vi "执行结果反馈与日志存储.vi"(9 "日志信息":string, 10 "error out":T1, 11 "设备":string) -> ()   [LabVIEW 2016]
panel:
  out "执行结果定义":u16(ring) items=["执行成功"=1, "执行失败，但不知道原因"=2, "命令请求条件错误"=3, "通讯超时"=4, "系统繁忙不能执行"=5, "系统故障"=6, "没有数据"=100]
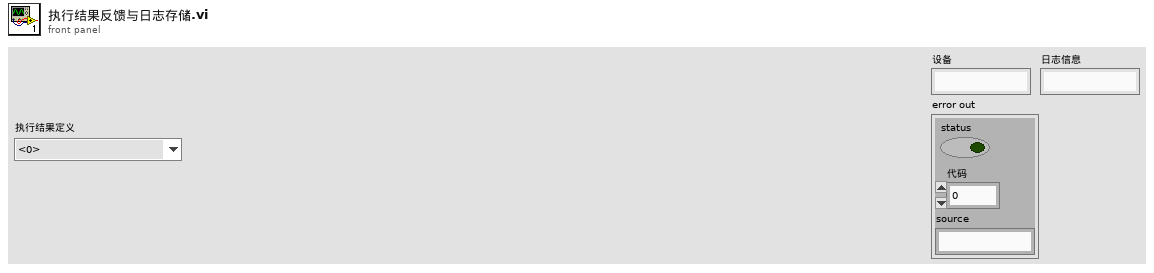
[diagram p1: front panel]
types:
  T1 = cluster{"status":bool, "代码":u16, "source":string}
  T2 = cluster{"时间标识":timestamp, "设备":string, "日志信息":string, "流程参数":string}
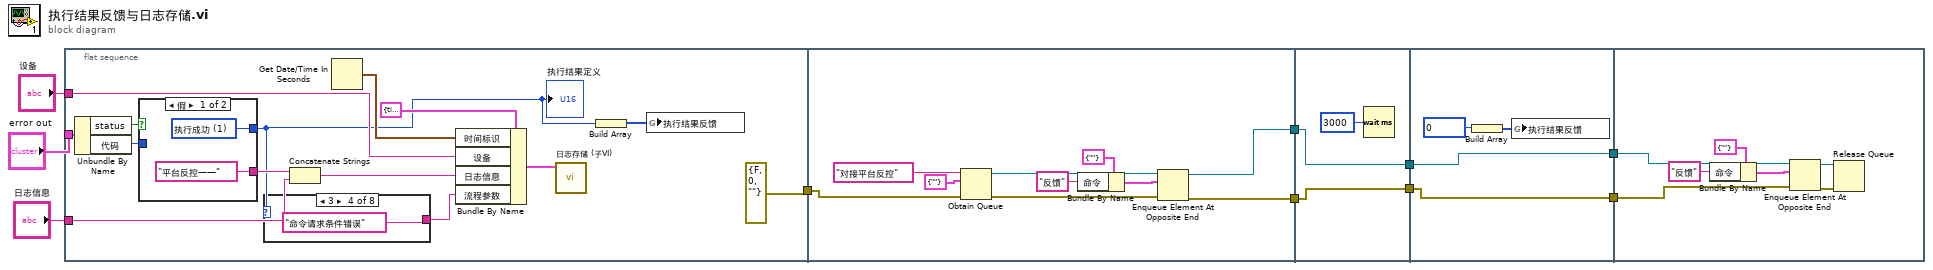
[diagram p0: block diagram]
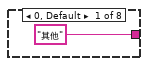
[diagram p2: hidden frame]
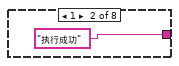
[diagram p3: hidden frame]
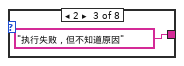
[diagram p4: hidden frame]
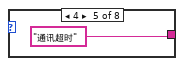
[diagram p5: hidden frame]
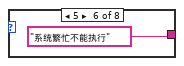
[diagram p6: hidden frame]
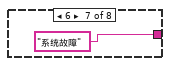
[diagram p7: hidden frame]
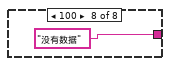
[diagram p8: hidden frame]
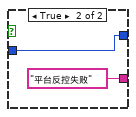
[diagram p9: hidden frame]
diagram:
  n1 = flat-sequence {
    tunnel: "日志信息" -> [w17]
    tunnel: "error out" -> [w16]
    tunnel: "设备" -> [w15]
    tunnel: [errorcluster {"status"=FALSE, "code"=0, "source"=""} ("错误输出")] -> w10
    tunnel: w10 -> [w39]
    tunnel: [w38] -> w9
    tunnel: [w37] -> w8
    tunnel: w9 -> [w49]
    tunnel: w8 -> [w48]
    tunnel: [w49] -> w7
    tunnel: [w48] -> w6
    tunnel: w7 -> [w51]
    tunnel: w6 -> [w50]
    tunnel: [w51] -> w5
    tunnel: [w50] -> w4
    tunnel: w5 -> [w57]
    tunnel: w4 -> [w56]
    frame #0 {
      n2 = Unbundle By Name(w16) -> ("status"=w23:bool, "代码"=w24:u16)
      n3 = case shown="假" w23 {
        tunnel: ["平台反控——" ("日志信息") "平台反控失败" ("日志信息")] -> w22
        tunnel: [w33 w35] -> w12
        tunnel: w24 -> [_ w35]
        frame False {
          w33 = u16 1 items=["执行成功"=1, "执行失败，但不知道原因"=2, "命令请求条件错误"=3, "通讯超时"=4, "系统繁忙不能执行"=5, "系统故障"=6, "没有数据"=100] ("执行结果定义")
        }
        frame True {
        }
      }
      "执行结果定义" <- w12
      n4 = case shown="3" w12 {
        tunnel: ["其他" "执行成功" "执行失败，但不知道原因" "命令请求条件错误" "通讯超时" "系统繁忙不能执行" "系统故障" "没有数据"] -> w11
        frame 0, Default {
        }
        frame 1 {
        }
        frame 2 {
        }
        frame 3 {
        }
        frame 4 {
        }
        frame 5 {
        }
        frame 6 {
        }
        frame 100 {
        }
      }
      n5 = Concatenate Strings(w22, w17) -> (w21:string)
      n6 = Get Date/Time In Seconds() -> (seconds since 1Jan1904=w18:timestamp)
      n7 = Bundle By Name(cluster=T2 {"时间标识"=timestamp(0 s since 1904-01-01), "设备"="", "日志信息"="", "流程参数"=""} ("data in"), "时间标识"=w18, "设备"=w15, "日志信息"=w21, "流程参数"=w11) -> (w19:T2)
      n8 = call "日志存储 (子VI).vi"("data in"=w19) -> ()  [unwired: 11 in]
      n9 = Build Array(w12) -> (w14:u16[])
      n10 = global write "modbus slave全局.vi" "执行结果反馈"(w14) -> ()
    }
    frame #1 {
      n11 = Obtain Queue(name (unnamed)="对接平台反控" ("名称（未命名）"), element data type=cluster{"命令":string} {"命令"=""}, error in (no error)=w39) -> (queue out=w44:refnum<queue>, error out=w43:errorcluster)  [unwired: 2 in, 1 out]
      n12 = Bundle By Name(cluster=cluster{"命令":string} {"命令"=""} ("元素"), "命令"="反馈") -> (w40:cluster{"命令":string})
      n13 = Enqueue Element At Opposite End(queue=w44, element=w40, error in (no error)=w43) -> (queue out=w38:refnum<queue>, error out=w37:errorcluster)  [unwired: 1 in, 1 out]
    }
    frame #2 {
      n14 = Wait (ms)(milliseconds to wait=u32 3000 ("等待时间（毫秒）")) -> ()  [unwired: 1 out]
    }
    frame #3 {
      w52 = u16 0 items=["执行成功"=1, "执行失败，但不知道原因"=2, "命令请求条件错误"=3, "通讯超时"=4, "系统繁忙不能执行"=5, "系统故障"=6, "没有数据"=100] ("执行结果定义")
      n15 = Build Array(w52) -> (w53:u16[])
      n16 = global write "modbus slave全局.vi" "执行结果反馈"(w53) -> ()
    }
    frame #4 {
      n17 = Bundle By Name(cluster=cluster{"命令":string} {"命令"=""} ("元素"), "命令"="反馈") -> (w58:cluster{"命令":string})
      n18 = Enqueue Element At Opposite End(queue=w57, element=w58, error in (no error)=w56) -> (queue out=w55:refnum<queue>, error out=w54:errorcluster)  [unwired: 1 in, 1 out]
      n19 = Release Queue(queue=w55, error in (no error)=w54) -> ()  [unwired: 1 in, 3 out]
    }
  }
